vi "Simulated EMG Example 2012.vi"(8 "error in (no error)":errorcluster) -> (0 "error out":errorcluster)   [LabVIEW 2012]
uses:
  <vilib>/addons/Biomedical/NI_BMTK_Measurements.lvlib
  <vilib>/addons/Biomedical/Biosignal Measurements/EMG/EMG Mean Power Frequency (Waveform).vi
panel:
  out "MNF":cluster{"t0":dbl, "dt":dbl, "frequency":dbl[]}(graph)
  in  "Stop":bool
  out "Simulated EMG Measurement":dynamicdata(graph)
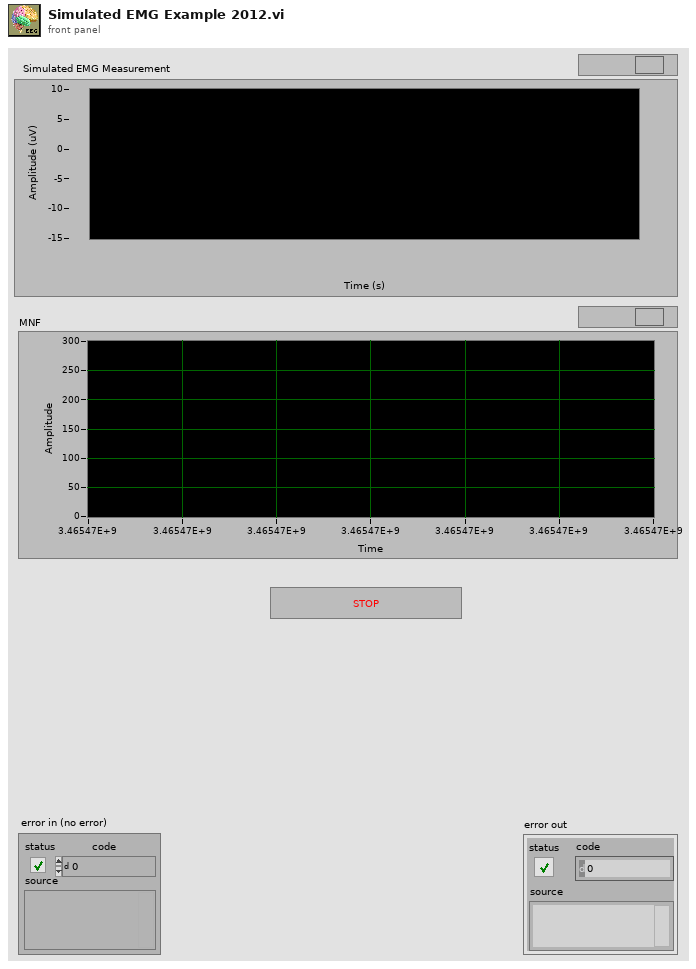
[diagram p1: front panel]
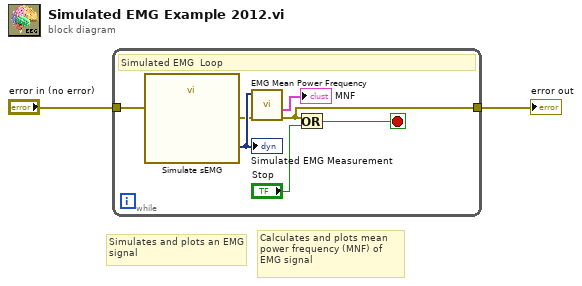
[diagram p0: block diagram]
diagram:
  # "Simulates and plots an EMG signal"
  # "Calculates and plots mean power frequency (MNF) of EMG signal"
  n1 = while {
    tunnel: "error in (no error)" -> [w7]
    tunnel: [w3] -> w1
    stop <- w9 stop-if-true
    # "Simulated EMG  Loop"
    n2 = call "Simulate sEMG"("error in (no error)"=w7) -> ("error out"=w4:errorcluster, "EMG"=w5:dynamicdata)  [unwired: 9 in]
    "Simulated EMG Measurement" <- w5
    n3 = call-poly <vilib>:"EMG Mean Power Frequency.vi"("error in (no error)"=w4, "EMG"=w5) -> ("error out"=w3:errorcluster, "MNF"=→"MNF":cluster{"t0":dbl, "dt":dbl, "frequency":dbl[]})  [unwired: 6 in, 2 out]
    n4 = Or(x=w3, y="Stop") -> (x .or. y?=w9:bool)
  }
  "error out" <- w1
